vi "SD Module_Initialize.vi"(7 "Module Model":T1, 8 "error in (no error)":errorcluster, 9 "Slot Settings":T4, 10 "Channels":T2={"# Input Channels"=0, "# Output Channels"=0, "Channel Type"=enum."Digital", "Units"=""}, 11 "SD Module in":refnum<class "SD Module.lvclass">) -> (0 "error out":errorcluster, 3 "SD Module out":refnum<class "SD Module.lvclass">)   [LabVIEW 2011, in "Modules.lvlib" / "SD Module.lvclass"]
uses:
  SD Module.lvclass
  RSI Module/Slot Settings.ctl
  RSI Module/Channels.ctl
  RSI Module/Channel Type.ctl
  RSI Module/Module Models.ctl
  SD Module.lvclass/SD Module.ctl
  RSI Module/RSI Module.lvclass
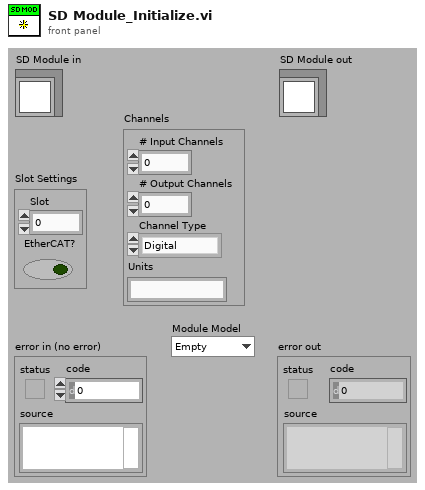
[diagram p1: front panel]
types:
  T1 = typedef "Modules.lvlib/RSI Module.lvclass/Module Models.ctl" = enum16{"Empty", "NI 9201", "NI 9203", "NI 9205", "NI 9206", "NI 9207", "NI 9208", "NI 9211", "NI 9213", "NI 9214", "NI 9215", "NI 9217", "NI 9219", "NI 9221", "NI 9225", "NI 9227", "NI 9229", "NI 9233", "NI 9234", "NI 9235", "NI 9236", "NI 9237", "NI 9239", "NI 9263", "NI 9264", "NI 9265", "NI 9269", "NI 9375", "NI 9401", "NI 9402", "NI 9403", "NI 9411", "NI 9421", "NI 9422", "NI 9423", "NI 9425", "NI 9426", "NI 9435", "NI 9472", "NI 9474", "NI 9475", "NI 9476", "NI 9477", "NI 9478", "NI 9481", "NI 9485"}
  T2 = typedef "Modules.lvlib/RSI Module.lvclass/Channels.ctl" = cluster{"# Input Channels":i32, "# Output Channels":i32, "Channel Type":T3, "Units":string}
  T3 = typedef "Modules.lvlib/RSI Module.lvclass/Channel Type.ctl" = enum16{"Analog", "Digital"}
  T4 = typedef "Modules.lvlib/RSI Module.lvclass/Slot Settings.ctl" = cluster{"Slot":u32, "EtherCAT?":bool}
  T5 = typedef "Modules.lvlib/SD Module.lvclass/Counter.ctl" = cluster{"Counter Channels":T6[]}
  T6 = typedef "Modules.lvlib/SD Module.lvclass/Counter Channel.ctl" = cluster{"Measurement Mode":u32, "Count Edges":T7, "Period Measurement":T8, "Pulse Width Measurement":T9, "Frequency Measurement":T10}
  T7 = typedef "Modules.lvlib/SD Module.lvclass/Count Edges.ctl" = cluster{"Counter Event":u32, "Counter Source":u32, "Counter Direction":u32, "Terminal Count":u32, "Output Mode":u32, "Gate Mode":u32}
  T8 = typedef "Modules.lvlib/SD Module.lvclass/Period Measurement.ctl" = cluster{"Measurement Edge":u32}
  T9 = typedef "Modules.lvlib/SD Module.lvclass/Pulse Width Measurement.ctl" = cluster{"Measurement Type":u32}
  T10 = typedef "Modules.lvlib/SD Module.lvclass/Frequency Measurement.ctl" = cluster{"Measurement Edge":u32, "Measurement Timebase":u32}
  T11 = typedef "Modules.lvlib/SD Module.lvclass/Quadrature.ctl" = cluster{"Quadrature Channels":T12[]}
  T12 = typedef "Modules.lvlib/SD Module.lvclass/Quadrature Channel.ctl" = cluster{"Timebase":u32, "Index Mode":u32}
  T13 = typedef "Modules.lvlib/SD Module.lvclass/CDO.ctl" = cluster{"Drive From Slot":u32, "CDO Channels":T14[]}
  T14 = typedef "Modules.lvlib/SD Module.lvclass/CDO Channel.ctl" = cluster{"Counter driven enabled":bool}
  T15 = typedef "Modules.lvlib/SD Module.lvclass/PWM.ctl" = cluster{"PWM Channels":T16[]}
  T16 = typedef "Modules.lvlib/SD Module.lvclass/PWM Channel.ctl" = cluster{"PWM frequency":u32}
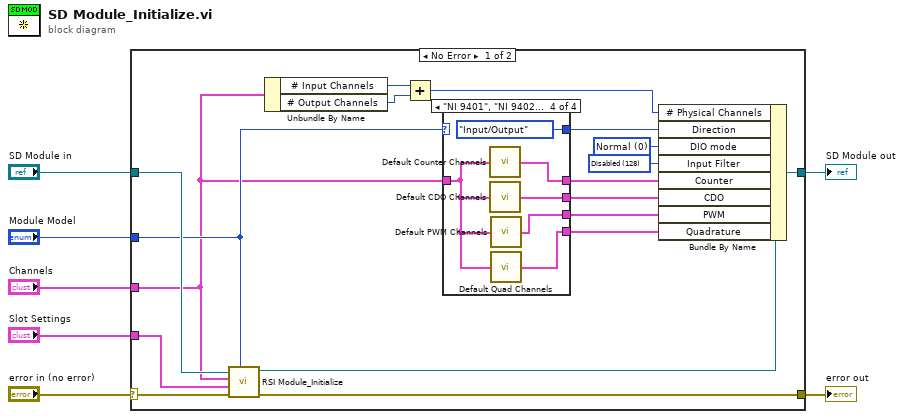
[diagram p0: block diagram]
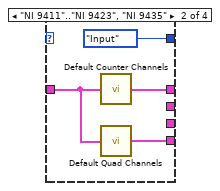
[diagram p3: hidden frame]
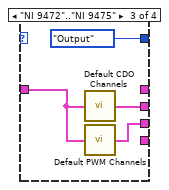
[diagram p4: hidden frame]
diagram:
  n1 = case shown="No Error" "error in (no error)" {
    selector: "error in (no error)" -> [w23 w41]
    tunnel: [w22 w41] -> w6
    tunnel: [w20 w40] -> w4
    tunnel: "SD Module in" -> [w25 w40]
    tunnel: "Slot Settings" -> [w24 _]
    tunnel: "Channels" -> [w11 _]
    tunnel: "Module Model" -> [w19 _]
    frame No Error {
      w16 = u32 128 items=["1 us"=0, "16 us"=1, "256 us"=2, "4096 us"=3, "Disabled"=128] ("Input Filter")
      w17 = u32 0 items=["Normal", "Counter", "Counter Slave", "PWM", "Quadrature"] ("DIO mode")
      n2 = call "RSI Module_Initialize.vi"("Module Model"=w19, "error in (no error)"=w23, "Slot Settings"=w24, "Channels"=w11, "RSI Module in"=w25) -> ("error out"=w22:errorcluster, "RSI Module out"=w21:refnum<class "SD Module.lvclass">)  [unwired: 5 in]
      n3 = Unbundle By Name(w11) -> ("# Input Channels"=w10:i32, "# Output Channels"=w9:i32)
      n4 = Add(x=w10, y=w9) -> (x+y=w8:i32)
      n5 = case shown="\"NI 9401\", \"NI 9402\"" w19 {
        tunnel: [_ enum16{"Input", "Output", "Input/Output"}."Input" ("Direction") enum16{"Input", "Output", "Input/Output"}."Output" ("Direction") enum16{"Input", "Output", "Input/Output"}."Input/Output" ("Direction")] -> w18
        tunnel: [_ w28 _ w38] -> w15
        tunnel: w11 -> [_ w26 w30 w35]
        tunnel: [_ _ w32 w37] -> w14
        tunnel: [_ _ w31 w36] -> w13
        tunnel: [_ w27 _ w34] -> w12
        frame "Empty", Default {
        }
        frame "NI 9411".."NI 9423", "NI 9435" {
          n6 = call "Default Counter Channels.vi"("Channels"=w26) -> ("Counter"=w28:T5)
          n7 = call "Default Quad Channels.vi"("Channels"=w26) -> ("Quadrature"=w27:T11)
        }
        frame "NI 9472".."NI 9475" {
          n8 = call "Default CDO Channels.vi"("Channels"=w30) -> ("CDO"=w32:T13)
          n9 = call "Default PWM Channels.vi"("Channels"=w30) -> ("PWM"=w31:T15)
        }
        frame "NI 9401", "NI 9402" {
          n10 = call "Default Counter Channels.vi"("Channels"=w35) -> ("Counter"=w38:T5)
          n11 = call "Default CDO Channels.vi"("Channels"=w35) -> ("CDO"=w37:T13)
          n12 = call "Default PWM Channels.vi"("Channels"=w35) -> ("PWM"=w36:T15)
          n13 = call "Default Quad Channels.vi"("Channels"=w35) -> ("Quadrature"=w34:T11)
        }
      }
      n14 = Bundle By Name(cluster=w21, "# Physical Channels"=w8, "Direction"=w18, "DIO mode"=w17, "Input Filter"=w16, "Counter"=w15, "CDO"=w14, "PWM"=w13, "Quadrature"=w12) -> (w20:refnum<class "SD Module.lvclass">)
    }
    frame Error {
    }
  }
  "error out" <- w6
  "SD Module out" <- w4
